vi "Search And Remove ID Priv.vi"(4 "Remove String":string, 5 "Strings In":string[](array[string])) -> (2 "Strings Out":string[](array[string]))   [LabVIEW 2020, in "NI_VIAnCFGDataStructure.lvlib" / "Tree.lvclass"]
uses:
  <vilib>/addons/analyzer/VIAnCFGDataStructure/Tree Manager/Tree.lvclass
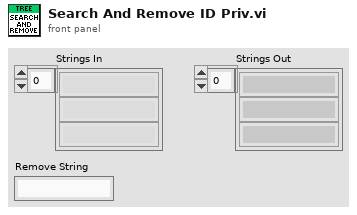
[diagram p1: front panel]
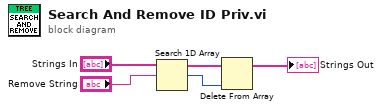
[diagram p0: block diagram]
diagram:
  n1 = Search 1D Array(1D array="Strings In", element="Remove String") -> (index of element=w2:i32)  [unwired: 1 in]
  n2 = Delete From Array(array="Strings In", index=w2) -> (array with subset deleted=→"Strings Out":string[])  [unwired: 1 in, 1 out]
